vi "onIncomingPacket.vi"(10 "ControlPacket":refnum<class "ControlPacket.lvclass">, 11 "PacketTracer in":refnum<class "PacketTracer.lvclass">) -> ()   [LabVIEW 2013, in "MQTT Server.lvlib" / "PacketTracer.lvclass"]
uses:
  PacketTracer.lvclass
  <vilib>/LabVIEW Open Source Project/MQTT Control Packets/Control Packets/ControlPacket/ControlPacket.lvclass
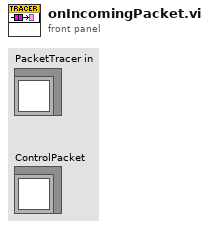
[diagram p1: front panel]
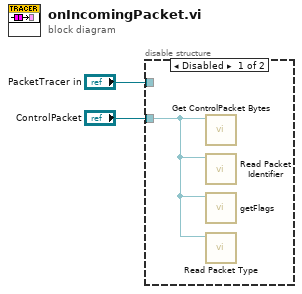
[diagram p0: block diagram]
diagram:
  n1 = disable-structure shown="Disabled" {
    disable-tunnel: "ControlPacket" -> [w3 _]
    disable-tunnel: "PacketTracer in" -> [_ _]
    frame Disabled {
      n2 = call <vilib>:"Get ControlPacket Bytes.vi"("ControlPacket"=w3) -> ()  [unwired: 7 in, 4 out]
      n3 = call <vilib>:"Read Packet Identifier.vi"("ControlPacket in"=w3) -> ()  [unwired: 9 in, 2 out]
      n4 = call-dynamic "getFlags.vi"("ControlPacket in"=w3) -> ()  [unwired: 7 in, 4 out]
      n5 = call <vilib>:"Read Packet Type.vi"("ControlPacket in"=w3) -> ()  [unwired: 9 in, 2 out]
    }
    frame Enabled {
    }
  }
